vi "LoadFPGA测试.vi"() -> ()   [LabVIEW 2011]
panel:
  in  "频率":dbl=1.0
  in  "设备资源名称":string="PXI4::2::INSTR"
  out "错误输出":errorcluster
  in  "FPGA文件":string="D:\\\\bit\\\\da_test.bit"
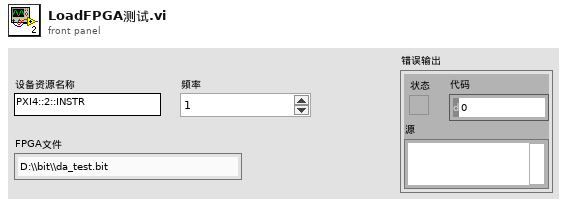
[diagram p1: front panel]
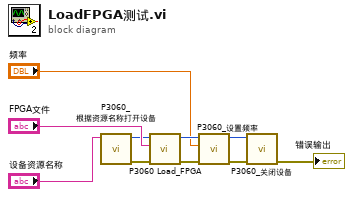
[diagram p0: block diagram]
diagram:
  n1 = call "P3060_根据资源名称打开设备.vi"("设备资源名称"="设备资源名称") -> ("error out"=w7:errorcluster, "句柄输出"=w9:i32)  [unwired: 9 in]
  n2 = call "P3060 Load_FPGA.vi"("错误输入（无错误）"=w7, "FPGA文件"="FPGA文件", "句柄输出"=w9) -> ("错误输出"=w4:errorcluster, "设备名"=w5:i32)  [unwired: 7 in]
  n3 = call "P3060_设置频率.vi"("错误输入"=w4, "频率"="频率", "句柄输入"=w5) -> ("错误输出"=w1:errorcluster, "句柄输出"=w2:i32)  [unwired: 6 in, 1 out]
  n4 = call "P3060_关闭设备.vi"("error in (no error)"=w1, "句柄输入"=w2) -> ("error out"=→"错误输出":errorcluster)  [unwired: 9 in]
